vi "ProcImageHD_DBL.vi"(7 "T/R Ring":i32, 8 "Scan Data In":i8[][](array[numeric]), 9 "Att (dB)":dbl) -> (0 "Synth App Out":i16[][](array[numeric]), 4 "Focal lengths":sgl[](array[numeric])=[0.0085, 0.009, 0.0095, 0.01, 0.0105, 0.011, 0.0115, 0.012, 0.0125, 0.013, 0.0135, 0.014, 0.0145, 0.015])   [LabVIEW 2022 SP3]
uses:
  ScanningControl/Motion Controllers/-MotionRoutines/MotionGlobals.vi
  <vilib>/Analysis/NI_AALBase.lvlib
  <vilib>/Analysis/baseanly.llb/Mean (DBL).vi
panel:
  in  "One Way Receive":bool
  in  "Type of Mean":u16(ring) items=["Mean from lines", "Mean just lines", "Poly Mean", "No mean"]
  in  "F3 20 MHz":dbl[](array[numeric])=[0.0, 0.0021173000000000003, 0.002217038688303391, 0.003063649156506908, 0.0031631091439381287, 0.0038030513383040436, 0.003902223261134889, 0.004435332245982045, 0.004534208485358321, 0.004999044189180914]
  in  "F2 40MHz":sgl[](array[numeric])=[0.0, 0.00132, 0.00142, 0.0019, 0.002, 0.00236, 0.00245, 0.00275, 0.00285, 0.0031]
  in  "Round to ROC?":bool
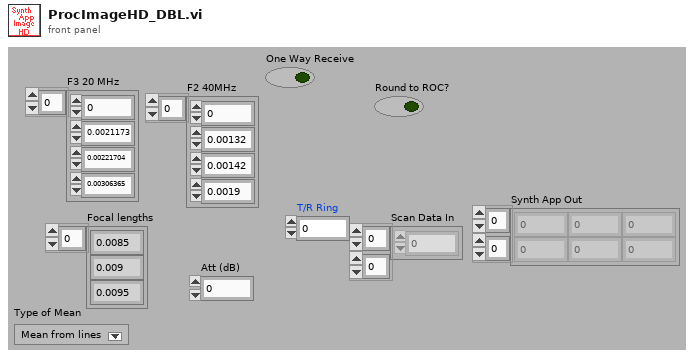
[diagram p1: front panel]
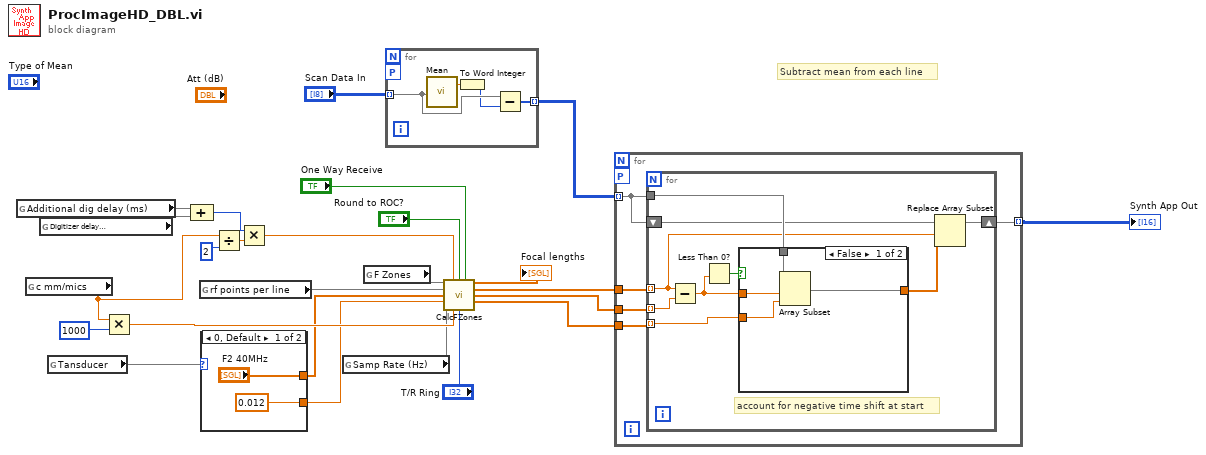
[diagram p0: block diagram]
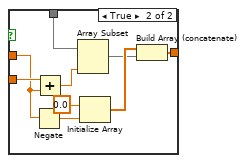
[diagram p2: hidden frame]
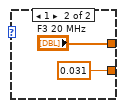
[diagram p3: hidden frame]
diagram:
  # "Subtract mean from each line"
  n1 = global read "MotionGlobals.vi" "Additional dig delay (ms)"() -> (w3)
  n2 = global read "MotionGlobals.vi" "c mm/mics"() -> (w9:sgl)
  n3 = global read "MotionGlobals.vi" "Digitizer delay\n (ms)"() -> (w2)
  n4 = global read "MotionGlobals.vi" "Tansducer"() -> (w18)
  n5 = Multiply(x=w9, y=1000) -> (x*y=w20:sgl)
  n6 = Compound Arithmetic op=ADD(w3, w2) -> (w1:i32)
  n7 = global read "MotionGlobals.vi" "rf points per line"() -> (w7)
  n8 = case shown="0, Default" w18 {
    tunnel: ["F2 40MHz" "F3 20 MHz"] -> w17
    tunnel: [0.012 ("ROC (mm)") 0.031 ("ROC (mm)")] -> w16
    frame 0, Default {
    }
    frame 1 {
    }
  }
  n9 = Divide(x=w9, y=2) -> (x/y=w24:sgl)
  n10 = Multiply(x=w1, y=w24) -> (x*y=w8:sgl)
  n11 = global read "MotionGlobals.vi" "Samp Rate (Hz)"() -> (w15)
  n12 = global read "MotionGlobals.vi" "F Zones"() -> (w23)
  n13 = for {
    tunnel: "Scan Data In" -> [w33] mode=indexing
    tunnel: [w32] -> w10 mode=indexing
    workers-P: _ -> [_]
    n14 = call-poly <vilib>:"Mean.vi"("X"=w33) -> ("mean"=w31:dbl)  [unwired: 1 out]
    n15 = To Word Integer(number=w31) -> (16bit integer=w30:i16)
    n16 = Subtract(x=w33, y=w30) -> (x-y=w32:i16[])
  }
  n17 = call "CalcFZones.vi"("F- zones"=w23, "delay (mm)"=w8, "Round to ROC?"="Round to ROC?", "One Way Receive"="One Way Receive", "# rf points per line"=w7, "Radii (m)"=w17, "ROC (m)"=w16, "Sampling Rate"=w15, "c (m/s)"=w20, "File index number"="T/R Ring") -> ("FZones (m)"=→"Focal lengths":dbl[], "ZoneStart"=w4:sgl[], "ZoneShift"=w5:sgl[], "ZoneLength"=w6:sgl[])  [unwired: 2 out]
  n18 = for {
    tunnel: w10 -> [w38] mode=indexing
    tunnel: w4 -> [w37]
    tunnel: w5 -> [w36]
    tunnel: w6 -> [w35]
    workers-P: _ -> [_]
    tunnel: [w34] -> w12 mode=indexing
    n19 = for {
      tunnel: w37 -> [w40] mode=indexing
      tunnel: w35 -> [w47] mode=indexing
      tunnel: w36 -> [w46] mode=indexing
      tunnel: w38 -> [w43]
      shift-right: [w42] -> w34
      shift-left: w38 -> [w41]
      # "account for negative time shift at start"
      n20 = Subtract(x=w40, y=w46) -> (x-y=w44:sgl)
      n21 = Less Than 0?(x=w44) -> (x < 0?=w45:bool)
      n22 = case shown="False" w45 {
        tunnel: w43 -> [w51 w59]
        tunnel: w47 -> [w49 w60]
        tunnel: [w50 w54] -> w39
        tunnel: w44 -> [w48 w57]
        frame False {
          n23 = Array Subset(array=w51, index=w48, length=w49) -> (w50:i16[])
        }
        frame True {
          n24 = Negate(x=w57) -> (-x=w52:sgl)
          n25 = Add(x=w60, y=w57) -> (x+y=w53:sgl)
          n26 = Array Subset(array=w59, length=w53) -> (w55:i16[])  [unwired: 1 in]
          n27 = Initialize Array(0.0, w52) -> (w56:dbl[])
          n28 = Build Array (concatenate)(w56, w55) -> (w54:dbl[])
        }
      }
      n29 = Replace Array Subset(array=w41, new element=w39, index=w40) -> (w42:i16[])
    }
  }
  "Synth App Out" <- w12
